vi "savePostProData.vi"(1 "display write dialog?":bool, 2 "append to file?":bool, 3 "Block Timing":T1) -> (0 "error out":errorcluster)   [LabVIEW 2017]
uses:
  Controls/blockTiming.ctl
  Globals/measurementGlobal.vi
panel:
  out "File Status":string="File not appended"
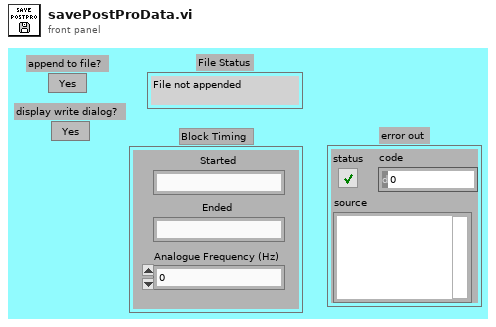
[diagram p1: front panel]
types:
  T1 = typedef "blockTiming.ctl" = cluster{"Started":string, "Ended":string, "Analogue Frequency (Hz)":dbl}
  T2 = typedef "postProData.ctl" = cluster{"Channel":string, "Samples":i32, "U":dbl, "u^2":dbl, "u^3":dbl, "u^4":dbl, "Kurtosis":dbl, "Skewness":dbl, "Turb":dbl}
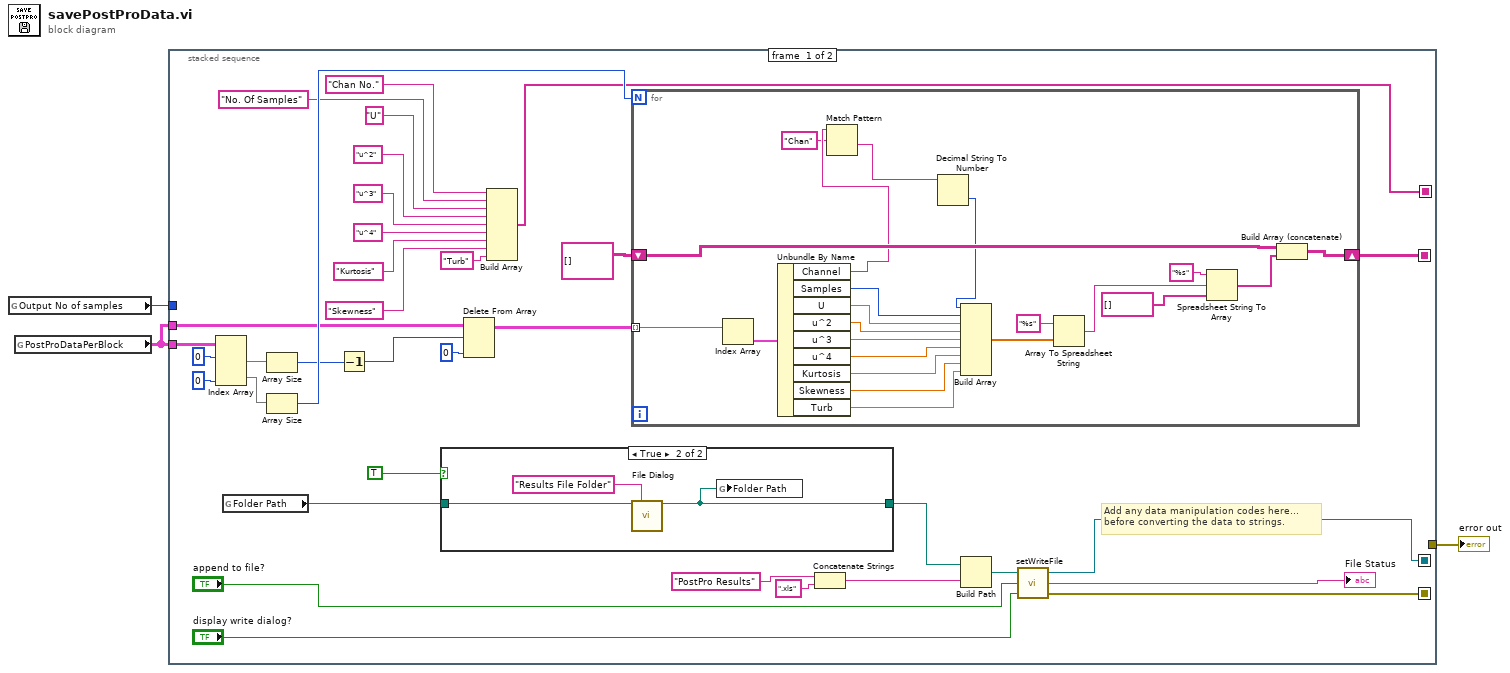
[diagram p0: block diagram]
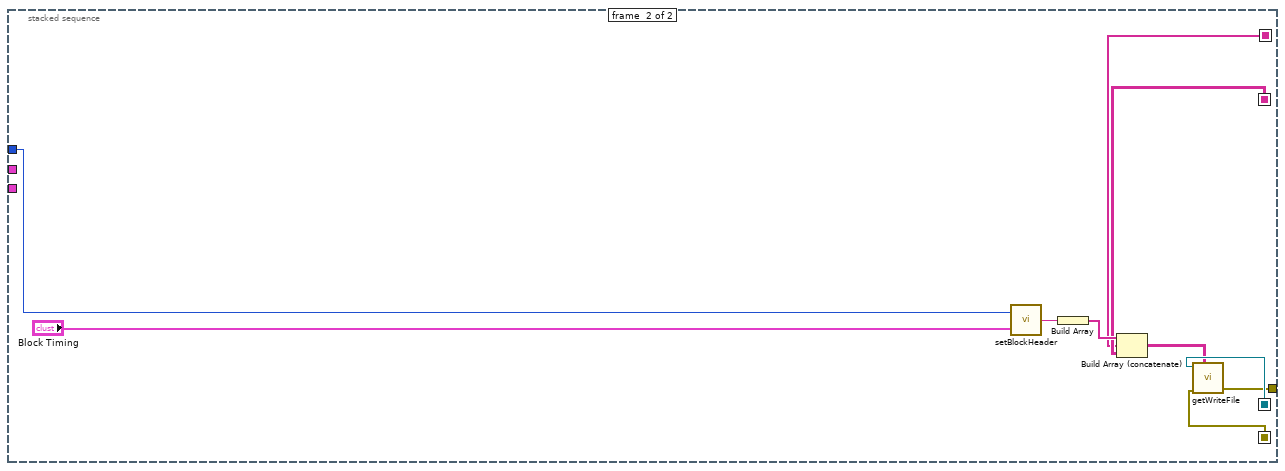
[diagram p3: hidden frame]
diagram:
  n1 = global read "measurementGlobal.vi" "Output No of samples"() -> (w3:i32)
  n2 = global read "measurementGlobal.vi" "PostProDataPerBlock"() -> (w1:T2[][])
  n3 = stacked-sequence {
    seq-local: [w36 _] -> [_ w70]
    seq-local: [w35 _] -> [_ w69]
    seq-local: [w17 _] -> [_ w66]
    seq-local: [w4 _] -> [_ w65]
    tunnel: w3 -> [_ w74]
    tunnel: [_ w67] -> w2
    tunnel: w1 -> [w26 _]
    tunnel: w1 -> [w22 _]
    frame #0 {
      # "Add any data manipulation codes here... \nbefore converting the data to strings."
      n4 = Index Array(array=w26, index (row) #1=0 ("index (row)"), index (col) #2=0 ("disabled index (col)")) -> (element #1=w24:T2[], element #2=w18:T2[])  [unwired: 2 in]
      n5 = global read "measurementGlobal.vi" "Folder Path"() -> (w31:path)
      n6 = Array Size(array=w24) -> (size(s)=w23:i32)
      n7 = Array Size(array=w18) -> (size(s)=w28:i32)
      n8 = Decrement(x=w23) -> (x-1=w21:i32)
      n9 = case shown="True" TRUE {
        tunnel: w31 -> [w61 w64]
        tunnel: [w61 w62] -> w30
        frame False {
        }
        frame True {
          n10 = call "File Dialog"("start path"=w64, "prompt"="Results File Folder") -> ("selected path"=w62:path)  [unwired: 10 in, 3 out]
          n11 = global write "measurementGlobal.vi" "Folder Path"(w62) -> ()
        }
      }
      n12 = Delete From Array(array=w22, length=w21, index (col)=0 ("index (row)")) -> (array with subset deleted=w14:T2[][])  [unwired: 1 in, 1 out]
      n13 = Build Array("Chan No." ("element"), "No. Of Samples" ("string"), "U" ("string"), "u^2" ("string"), "u^3" ("string"), "u^4" ("string"), "Kurtosis" ("string"), "Skewness" ("string"), "Turb" ("string")) -> (w4:string[])
      n14 = for {
        N: w28 -> [_]
        tunnel: w14 -> [w60] mode=indexing
        shift-right: [w45] -> w17
        shift-left: string[][] [] -> [w46]
        n15 = Index Array(array=w60) -> (element=w59:T2)  [unwired: 1 in]
        n16 = Unbundle By Name(w59) -> ("Channel"=w42:string, "Samples"=w58:i32, "U"=w57:dbl, "u^2"=w56:dbl, "u^3"=w55:dbl, "u^4"=w54:dbl, "Kurtosis"=w53:dbl, "Skewness"=w52:dbl, "Turb"=w51:dbl)
        n17 = Match Pattern(string=w42, regular expression="Chan") -> (after substring=w40:string)  [unwired: 1 in, 3 out]
        n18 = Decimal String To Number(string=w40) -> (number=w39:i32)  [unwired: 2 in, 1 out]
        n19 = Build Array(w39, w58, w57, w56, w55, w54, w53, w52, w51) -> (w50:dbl[])
        n20 = Array To Spreadsheet String(array=w50, 3:"%s" ("format string")) -> (spreadsheet string=w49:string)  [unwired: 1 in]
        n21 = Spreadsheet String To Array(format string="%s", spreadsheet string=w49, array type (2D Dbl)=string[] []) -> (array=w44:string[])  [unwired: 1 in]
        n22 = Build Array (concatenate)(w46, w44) -> (w45:string[][])
      }
      n23 = Concatenate Strings("PostPro Results", ".xls") -> (w32:string)
      n24 = Build Path(base path=w30, name or relative path=w32) -> (appended path=w38:path)
      n25 = call "setWriteFile.vi"("display write dialog?"="display write dialog?", "append to file?"="append to file?", "file path"=w38) -> ("error out"=w35:errorcluster, "Status"=→"File Status":string, "File Refnum"=w36:refnum<file>)
    }
    frame #1 {
      n26 = call "setBlockHeader.vi"("Block Timing"="Block Timing", "No of Analog. Samples"=w74) -> ("Output String"=w72:string)
      n27 = Build Array(w72) -> (w71:string[])
      n28 = Build Array (concatenate)(w71, w65, w66) -> (w68:string[][])
      n29 = call "getWriteFile.vi"("refnum in"=w70, "error in"=w69, "Data"=w68) -> ("error out"=w67:errorcluster)  [unwired: 2 in, 2 out]
    }
  }
  "error out" <- w2
